vi "SubStage_OpenNewWorkSheet.vi"(2 "error in (no error)":errorcluster, 4 "Excel._Workbook":refnum<k7>) -> (0 "error out":errorcluster, 1 "Excel._Worksheet":refnum<k7>)   [LabVIEW 2015]
doc: "Opens a new WorkSheet. Takes a Workbook Refnum as input."
panel:
  in  "Excel._Worksheet":refnum<k7>
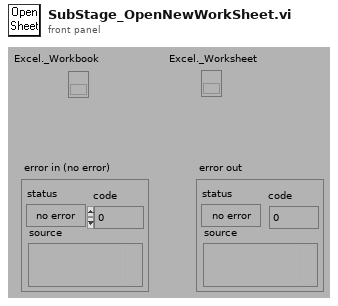
[diagram p1: front panel]
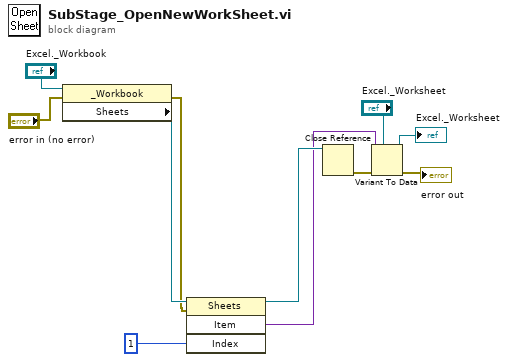
[diagram p0: block diagram]
diagram:
  n1 = property class="_Workbook"(reference="Excel._Workbook", error in="error in (no error)") -> (error out=w2:errorcluster, "Sheets"=w5:refnum<k7>)  [unwired: 1 out]
  n2 = invoke class="Sheets" method="Item"(reference=w5, error in=w2, "Index"=1) -> (reference out=w4:refnum<k7>, "Item"=w3:variant)  [unwired: 1 in, 2 out]
  n3 = Close Reference(reference=w4) -> (error out=w6:errorcluster)  [unwired: 1 in]
  n4 = Variant To Data(error in=w6, type="Excel._Worksheet", Variant=w3) -> (data=→"Excel._Worksheet":refnum<k7>, error out=→"error out":errorcluster)
